vi "Get ni_bus_monitor_api_StreamBusRequest.vi"(8 "error in (no error)":errorcluster, 11 "gRPCid":T1) -> (0 "error out":errorcluster, 2 "package_templatemessage":T2, 3 "gRPCid out":T1)   [LabVIEW 2025, in "bus_monitor_server.lvlib"]
uses:
  bus_monitor_server.lvlib
  ni_bus_monitor_api_StreamBusRequest.ctl
  ni_bus_monitor_api_Session.ctl
  <vilib>/gRPC/LabVIEW gRPC Library/Shared/grpcId.ctl
  ni_bus_monitor_api_StreamBusRequest_Flat.ctl
  ni_bus_monitor_api_Session_Flat.ctl
  2ed25e12-861d-4677-8ead-ace2906b2041.vi
  <vilib>/gRPC/LabVIEW gRPC Library/Shared/TranslateGrpcError.vi
  FlatToRichni_bus_monitor_api_Session.vi
  <vilib>/gRPC/LabVIEW gRPC Library/Server API/Server/Get Server DLL Path.vi
  <vilib>/Utility/error.llb/Error Cluster From Error Code.vi
  <vilib>/gRPC/LabVIEW gRPC Library/grpc-lvsupport-release.lvlib
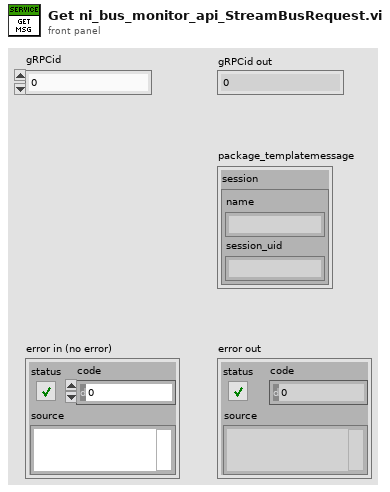
[diagram p1: front panel]
types:
  T1 = typedef "grpc-lvsupport-release.lvlib/grpcId.ctl" = u64
  T2 = typedef "bus_monitor_server.lvlib/ni_bus_monitor_api_StreamBusRequest.ctl" = cluster{"session":T3}
  T3 = typedef "bus_monitor_server.lvlib/ni_bus_monitor_api_Session.ctl" = cluster{"name":string, "session_uid":string}
  T4 = typedef "bus_monitor_server.lvlib/ni_bus_monitor_api_StreamBusRequest_Flat.ctl" = cluster{"session":T5}
  T5 = typedef "bus_monitor_server.lvlib/ni_bus_monitor_api_Session_Flat.ctl" = cluster{"name":string, "session_uid":string}
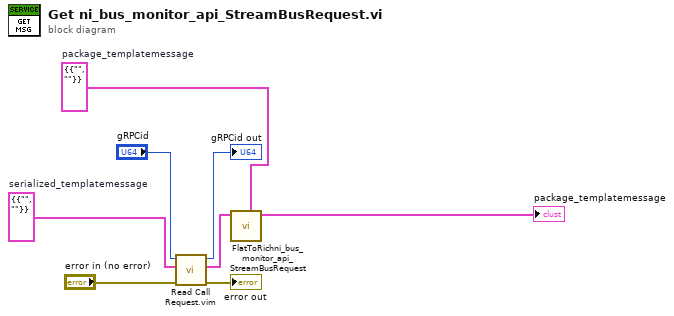
[diagram p0: block diagram]
diagram:
  w6 = T4 {"session"={"name"="", "session_uid"=""}}  # serialized_templatemessage
  w5 = T2 {"session"={"name"="", "session_uid"=""}}  # package_templatemessage
  n1 = call "Read Call Request.vim"("error in"="error in (no error)", "Request Type"=w6, "gRPCid in"="gRPCid") -> ("error out"=→"error out":errorcluster, "Request Data"=w4:T4, "gRPCid out"=→"gRPCid out":T1)  [unwired: 6 in]
  n2 = call "FlatToRichni_bus_monitor_api_StreamBusRequest.vi"("OutputClusterType"=w5, "InputCluster"=w4) -> ("OutputCluster"=→"package_templatemessage":T2)  [unwired: 9 in]
